vi "read_next_item.vi"(8 "error in (no error)":errorcluster, 9 "Wrap? (F)":bool, 11 "StringList in":refnum<class "StringList.lvclass">) -> (0 "error out":errorcluster, 1 "At Bottom?":bool, 2 "List Item":string, 3 "StringList out":refnum<class "StringList.lvclass">)   [LabVIEW 2015, in "StringList.lvlib" / "StringList.lvclass"]
uses:
  StringList.lvclass
  StringList.lvclass/StringList.ctl
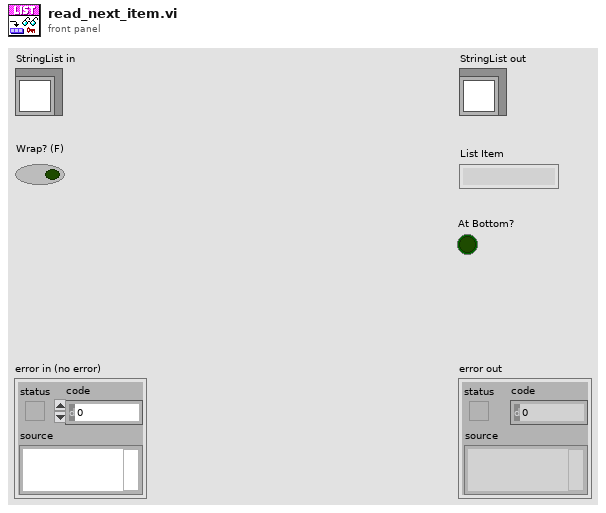
[diagram p1: front panel]
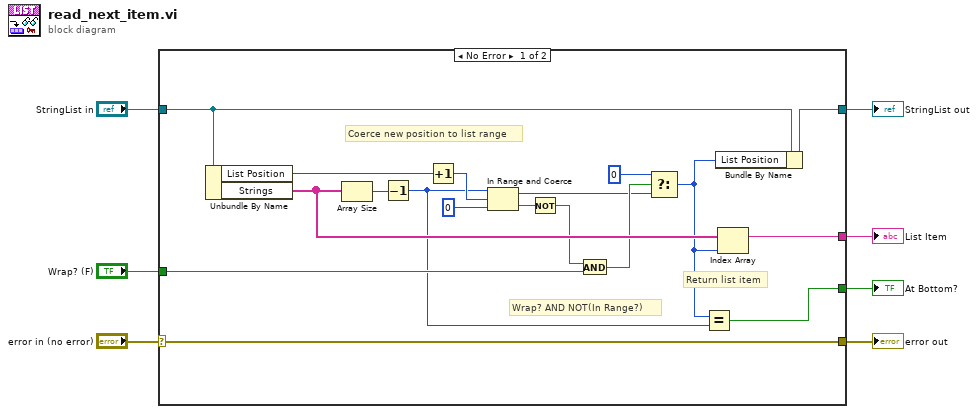
[diagram p0: block diagram]
diagram:
  n1 = case shown="No Error" "error in (no error)" {
    selector: "error in (no error)" -> [w25 w27]
    tunnel: [w25 w27] -> w6
    tunnel: [w22 w26] -> w4
    tunnel: "StringList in" -> [w24 w26]
    tunnel: [w23 _] -> w3
    tunnel: "Wrap? (F)" -> [w11 _]
    tunnel: [w8 _] -> w1
    frame No Error {
      # "Wrap? AND NOT(In Range?)"
      # "Coerce new position to list range"
      # "Return list item"
      n2 = Unbundle By Name(w24) -> ("List Position"=w21:i32, "Strings"=w20:string[])
      n3 = Array Size(array=w20) -> (size(s)=w18:i32)
      n4 = Decrement(x=w18) -> (x-1=w9:i32)
      n5 = Increment(x=w21) -> (x+1=w19:i32)
      n6 = In Range and Coerce(upper limit=w9, x=w19, lower limit=0) -> (coerced(x)=w13:i32, In Range?=w16:bool)
      n7 = Not(x=w16) -> (.not. x?=w15:bool)
      n8 = And(x=w15, y=w11) -> (x .and. y?=w14:bool)
      n9 = Select(t=0, s=w14, f=w13) -> (s? t:f=w10:i32)
      n10 = Equal?(x=w10, y=w9) -> (x = y?=w8:bool)
      n11 = Bundle By Name(cluster=w24, "List Position"=w10) -> (w22:refnum<class "StringList.lvclass">)
      n12 = Index Array(array=w20, index=w10) -> (element=w23:string)
    }
    frame Error {
    }
  }
  "error out" <- w6
  "StringList out" <- w4
  "List Item" <- w3
  "At Bottom?" <- w1
